vi "Initialize Rx Transfers.vi"(8 "error in (no error)":errorcluster, 9 "convert buffer":bool, 10 "Rx Transfer configurations":T2[](array[typedef]) {"channels"."string offset" format="%d bytes"}, 11 "UDP Transceiver in":refnum<class "UDP Transceiver.lvclass">) -> (0 "error out":errorcluster, 1 "max buffer size":u64, 2 "Rx Transfer parameters":T1[](array[typedef]) {"timeout" format="%d ms"}, 3 "UDP Transceiver out":refnum<class "UDP Transceiver.lvclass">)   [LabVIEW 2017, in "UDP.lvlib" / "UDP Transceiver.lvclass"]
uses:
  UDP Transceiver.lvclass
  Builds/Data Sharing Framework/Current/Core/DSF Core.lvlibp/Typedefs/DSF Engine Transfer Configuration.ctl
  Builds/Data Sharing Framework/Current/Core/DSF Core.lvlibp/Typedefs/DSF Byte Order.ctl
  Builds/Data Sharing Framework/Current/Core/DSF Core.lvlibp/Typedefs/DSF Settings Info.ctl
  Builds/Data Sharing Framework/Current/Core/DSF Core.lvlibp/Typedefs/DSF Engine Channel Configuration.ctl
  Builds/Data Sharing Framework/Current/Core/DSF Core.lvlibp/Typedefs/DSF Data Type.ctl
  Transfer Rx Parameters.ctl
  Builds/Data Sharing Framework/Current/Core/DSF Core.lvlibp/Classes/Configuration/Required Buffer Size (Transfer).vi
  UDP Invalid Setting.vi
  Builds/Data Sharing Framework/Current/Core/DSF Core.lvlibp/Classes/Configuration/Configuration Session.lvclass
  Builds/Data Sharing Framework/Current/Core/DSF Core.lvlibp
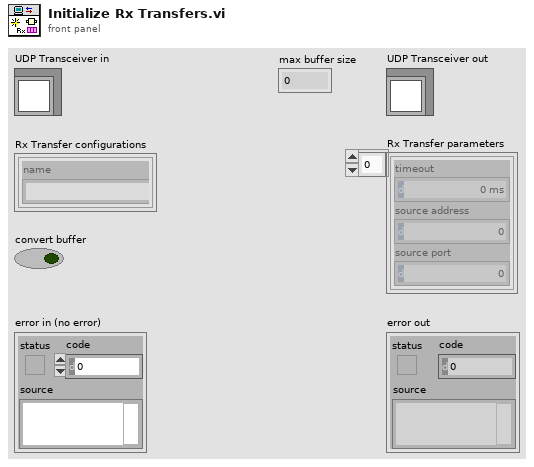
[diagram p1: front panel]
types:
  T1 = typedef "UDP.lvlib/UDP Transceiver.lvclass/Transfer Rx Parameters.ctl" = cluster{"timeout":i32, "source address":u32, "source port":u16}
  T2 = typedef "DSF Core.lvlibp/DSF Engine Transfer Configuration.ctl" = cluster{"name":string, "byte order":T3, "settings":T4, "channels":T5[]}
  T3 = typedef "DSF Core.lvlibp/DSF Byte Order.ctl" = enum8{"big-endian", "little-endian"}
  T4 = typedef "DSF Core.lvlibp/DSF Settings Info.ctl" = cluster{"component":string, "name":string, "values":cluster{"key":string, "value":string}[]}[]
  T5 = typedef "DSF Core.lvlibp/DSF Engine Channel Configuration.ctl" = cluster{"string offset":u64, "name":string, "units":string, "engine data type":T6, "string data type":T6, "settings":T4}
  T6 = typedef "DSF Core.lvlibp/DSF Data Type.ctl" = enum8{"Bool", "SGL", "DBL", "I8", "I16", "I32", "I64", "U8", "U16", "U32", "U64"}
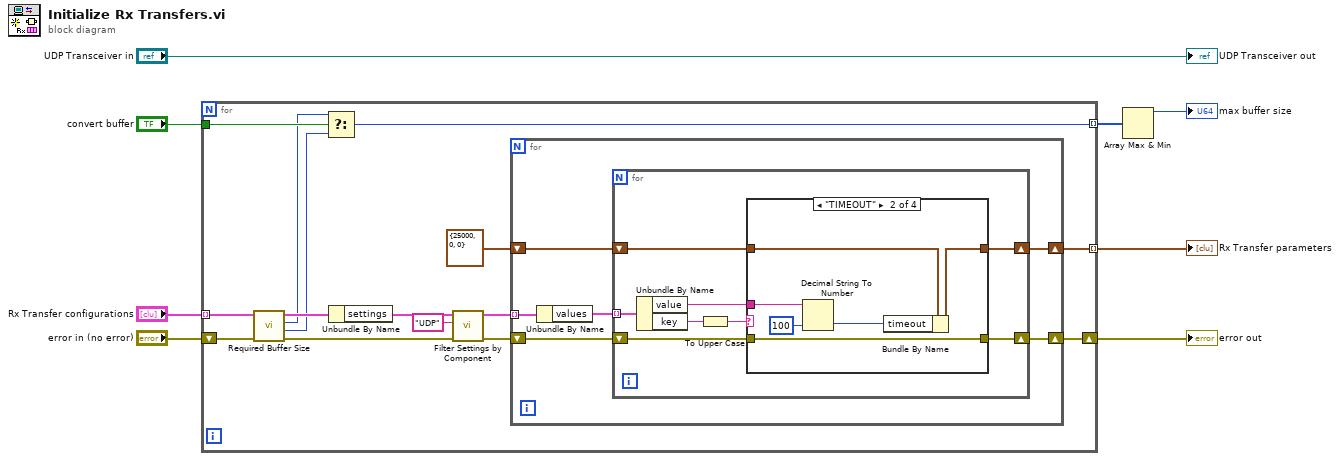
[diagram p0: block diagram]
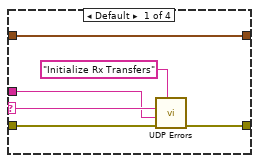
[diagram p2: hidden frame]
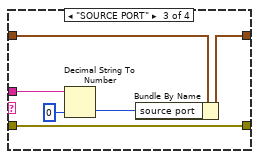
[diagram p3: hidden frame]
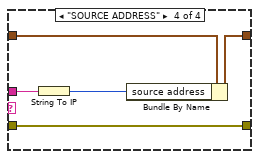
[diagram p4: hidden frame]
diagram:
  n1 = for {
    shift-right: [w23] -> w5
    shift-left: "error in (no error)" -> [w19]
    tunnel: "Rx Transfer configurations" -> [w20] mode=indexing
    tunnel: [w21] -> w6 mode=indexing
    tunnel: [w9] -> w4 mode=indexing
    tunnel: "convert buffer" -> [w12]
    n2 = call-poly "Required Buffer Size.vi"("error in (no error)"=w19, "Transfer Configuration in"=w20) -> ("error out"=w17:errorcluster, "engine buffer size"=w11:u64, "string buffer size"=w10:u64, "Transfer Configuration out"=w18:T2)  [unwired: 6 in]
    n3 = Select(t=w10, s=w12, f=w11) -> (s? t:f=w9:u64)
    n4 = Unbundle By Name(w18) -> ("settings"=w13:T4)
    n5 = call "Filter Settings by Component.vi"("error in (no error)"=w17, "component"="UDP", "settings"=w13) -> ("error out"=w16:errorcluster, "filtered settings"=w14:T4)  [unwired: 7 in]
    n6 = for {
      tunnel: w14 -> [w25] mode=indexing
      shift-right: [w27] -> w21
      shift-left: T1 {"timeout"=25000, "source address"=0, "source port"=0} ("Transfer Rx") -> [w28]
      shift-right: [w29] -> w23
      shift-left: w16 -> [w26]
      n7 = Unbundle By Name(w25) -> ("values"=w24:cluster{"key":string, "value":string}[])
      n8 = for {
        tunnel: w24 -> [w34] mode=indexing
        shift-right: [w35] -> w29
        shift-left: w26 -> [w36]
        shift-right: [w33] -> w27
        shift-left: w28 -> [w32]
        n9 = Unbundle By Name(w34) -> ("value"=w31:string, "key"=w37:string)
        n10 = To Upper Case(1:w37) -> (0:w30:string)
        n11 = case shown="\"TIMEOUT\"" w30 {
          selector: w30 -> [w39 _ _ _]
          tunnel: w31 -> [w38 w49 w55 w57]
          tunnel: w36 -> [w42 w46 w52 w60]
          tunnel: [w41 w46 w52 w60] -> w35
          tunnel: w32 -> [w40 w45 w51 w59]
          tunnel: [w40 w44 w50 w58] -> w33
          frame Default {
            n12 = call-poly "UDP Errors.vi"("source vi name"="Initialize Rx Transfers", "error in (no error)"=w42, "value"=w38, "key"=w39) -> ("error out"=w41:errorcluster)  [unwired: 6 in, 1 out]
          }
          frame "TIMEOUT" {
            n13 = Decimal String To Number(string=w49, default (0L)=100 ("default (0 I32)")) -> (number=w47:i32)  [unwired: 1 in, 1 out]
            n14 = Bundle By Name(cluster=w45, "timeout"=w47) -> (w44:T1)
          }
          frame "SOURCE PORT" {
            n15 = Decimal String To Number(string=w55, default (0L)=u16 0 ("default (0 I32)")) -> (number=w53:u16)  [unwired: 1 in, 1 out]
            n16 = Bundle By Name(cluster=w51, "source port"=w53) -> (w50:T1)
          }
          frame "SOURCE ADDRESS" {
            n17 = String To IP(1:w57) -> (0:w56:u32)
            n18 = Bundle By Name(cluster=w59, "source address"=w56) -> (w58:T1)
          }
        }
      }
    }
  }
  "error out" <- w5
  "Rx Transfer parameters" <- w6
  n19 = Array Max & Min(array=w4) -> (max value=→"max buffer size":u64)  [unwired: 3 out]
  "UDP Transceiver out" <- "UDP Transceiver in"
